vi "List Index Write.vi"(4 "error in (no error)":errorcluster caption="错误输入（无错误）", 5 "Value":i32 caption="值", 6 "Container State":T2 caption="容器状态", 7 "Display State In":T1 caption="显示状态输入") -> (0 "error out":errorcluster caption="错误输出", 3 "Display State Out":T1 caption="显示状态输出")   [LabVIEW 2011, in "NISAST Include Paths.xctl"]
uses:
  NISAST Include Paths.xctl
  <vilib>/_xctls/Container State.ctl
  State.ctl
  <vilib>/_xctls/XControlSupport.lvlib
panel:
  # "将以下值显示控件替换为所需类型的显示控件。\n不要从连线板中删除该显示控件或其它显示控件。\n不要更改连线板模式。\n值显示控件应始终位于连线板输出端自顶部起第三个接线端。"
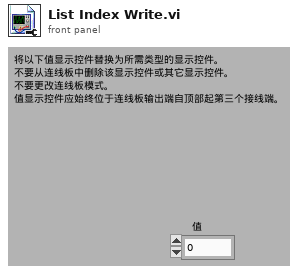
[diagram p1: front panel]
types:
  T1 = typedef "NISAST Include Paths.xctl/State.ctl" = cluster{"Edit Index":i32, "List Index":i32, "Label Text":string}
  T2 = typedef "XControlSupport.lvlib/Container State.ctl" = cluster{"Indicator?":bool, "Run Mode?":bool, " Refnum":refnum<vi>}
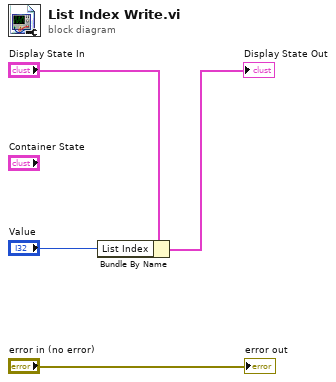
[diagram p0: block diagram]
diagram:
  n1 = Bundle By Name(cluster="Display State In", "List Index"="Value") -> (→"Display State Out":T1)
  "error out" <- "error in (no error)"
